vi "HMI-Malicious.vi"() -> ()   [LabVIEW 2017]
uses:
  <vilib>/Platform/TimedLoop/XDataNode/timing_clust.ctl
  <vilib>/Platform/TimedLoop/XDataNode/nitl_modes.ctl
  <vilib>/Platform/TimedLoop/XDataNode/wakeup.ctl
  <vilib>/Platform/TimedLoop/XDataNode/XDataNode.xnode
  <vilib>/Platform/TimedLoop/XDataNode/XDNodeRunTimeDep.lvlib
panel:
  in  "Transmitter port number":u16
  in  "Receiver Port number":u16
  in  "Receiver IP address":string
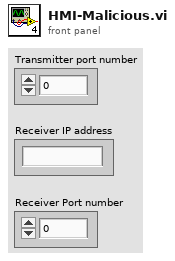
[diagram p1: front panel]
types:
  T1 = typedef "XDNodeRunTimeDep.lvlib/timing_clust.ctl" = cluster{"Expected End [f-1]":u64, "Actual End [f-1]":u64, "Finished Late? [f-1]":bool, "Expected End [i-1]":u64, "Actual End [i-1]":u64, "Finished Late? [i-1]":bool, "Expected Start [i]":u64, "Actual Start [i]":u64, "Expected Start [f]":u64, "Actual Start [f]":u64, "Source Name":string, "Structure Name":string, "Period":i64, "Deadline":i64, "Offset":i64, "Start":i64, "Priority":i32, "Timeout":i32, "Mode":T2, "Wakeup Reason":T3, "Error":errorcluster, "Source Type":string, "Secondary Source Type":string, "Global End Time":u64, "Global Start Time":u64, "Frame Duration":u64, "Iteration Duration":u64, "Assigned CPU":i32, "I/O Scan Engine Mode":u32}
  T2 = typedef "XDNodeRunTimeDep.lvlib/nitl_modes.ctl" = enum32{"No Change", "Process missed periods, maintain original phase", "Discard missed periods, maintain original phase", "Process missed periods, ignore original phase", "Discard missed periods, ignore original phase"}
  T3 = typedef "XDNodeRunTimeDep.lvlib/wakeup.ctl" = enum32{"Normal", "Aborted", "Asynchronous wakeup", "Timing source error", "Timed loop error", "Timeout"}
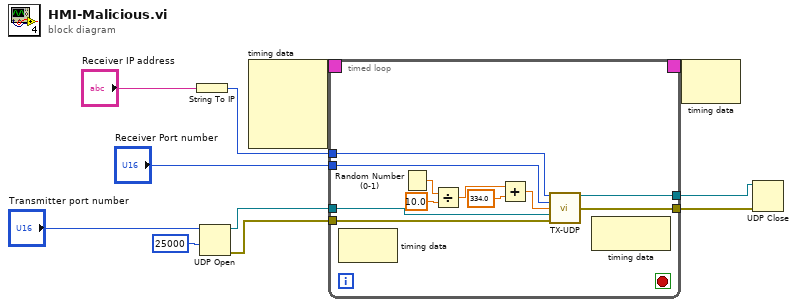
[diagram p0: block diagram]
diagram:
  n1 = String To IP(1:"Receiver IP address") -> (0:w10:u32)
  n2 = UDP Open(9:25000 ("timeout ms (25000)"), 11:"Transmitter port number") -> (port=w9:refnum<k16>, 0:w8:errorcluster)  [unwired: 3 in, 1 out]
  n3 = node-c288() -> (w5:T1)  [unwired: 4 in]
  n4 = timed-loop {
    tunnel: w10 -> [w18]
    tunnel: w9 -> [w17]
    tunnel: w8 -> [w16]
    tunnel: [w14] -> w7
    tunnel: [w13] -> w6
    timing: w5 -> [_]
    timing-out: [_] -> w4
    tunnel: "Receiver Port number" -> [w12]
    stop <- _ stop-if-true
    n5 = node-c288() -> ()  [unwired: 1 in, 1 out]
    n6 = Random Number (0-1)() -> (number: 0 to 1=w20:dbl)
    n7 = Divide(x=w20, y=10.0) -> (x/y=w19:dbl)
    n8 = Add(x=w19, y=334.0) -> (x+y=w15:dbl)
    n9 = call "TX-UDP.vi"("IP address"=w18, "Port number"=w12, "Data (Number)"=w15, "connection ID"=w17, "error in (no error)"=w16) -> ("connection ID out"=w13:refnum<k16>, "error out"=w14:errorcluster)  [unwired: 9 in]
    n10 = node-c288() -> ()  [unwired: 1 in, 1 out]
  }
  n11 = node-c288(w4) -> ()  [unwired: 1 out]
  n12 = UDP Close(connection ID=w6, 8:w7) -> ()  [unwired: 2 out]
